vi "ion pump controller.vi"() -> ()   [LabVIEW 2010]
panel:
  out "Pressure":cluster{dbl, dbl}[](graph)
  in  "TC or AC?":u16(ring) items=["AC", "TC"]
  out "Pressure (Torr)":dbl
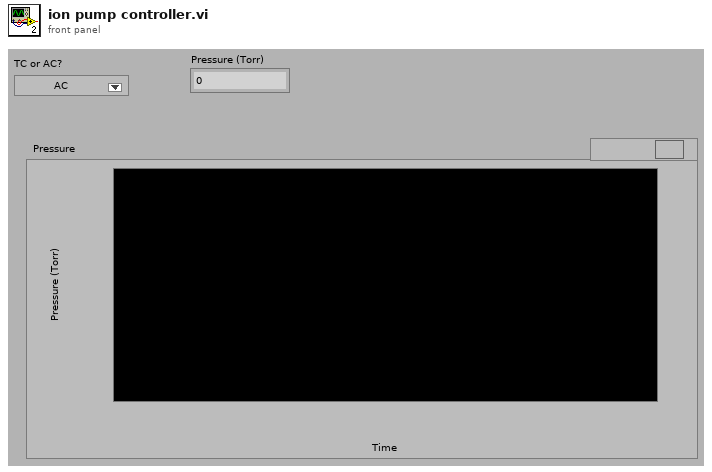
[diagram p1: front panel]
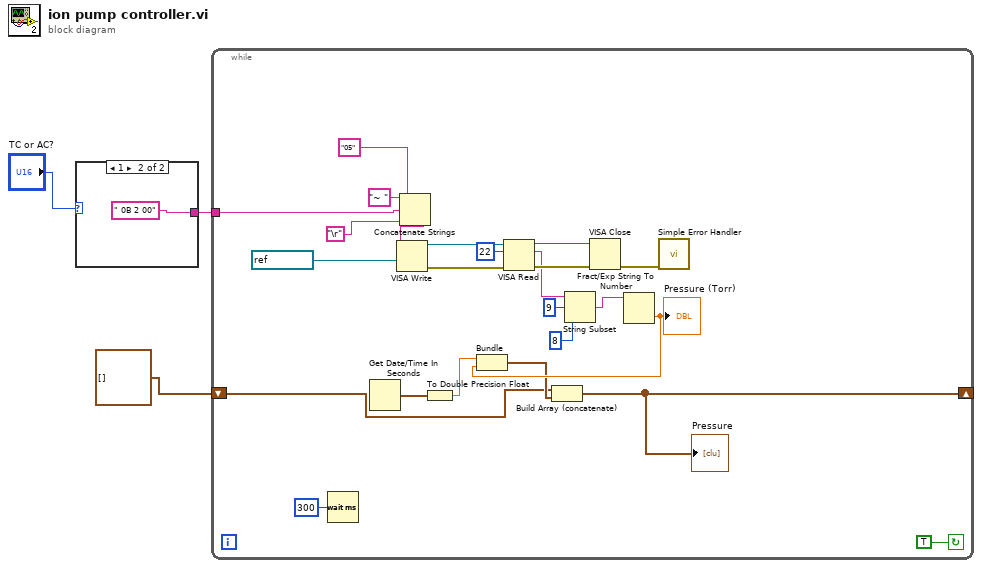
[diagram p0: block diagram]
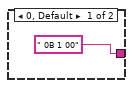
[diagram p2: hidden frame]
diagram:
  n1 = case shown="1" "TC or AC?" {
    tunnel: [" 0B 1 00" ("string") " 0B 2 00" ("string")] -> w3
    frame 0, Default {
    }
    frame 1 {
    }
  }
  n2 = while {
    tunnel: w3 -> [w18]
    shift-right: [w7] -> _
    shift-left: cluster{dbl, dbl}[] [] -> [w8]
    stop <- TRUE continue-if-true
    n3 = Wait (ms)(milliseconds to wait=u32 300) -> ()  [unwired: 1 out]
    n4 = Get Date/Time In Seconds() -> (seconds since 1Jan1904=w12:timestamp)
    n5 = Concatenate Strings("~ " ("string"), "05" ("string"), w18, "\r") -> (w29:string)
    n6 = VISA Write(VISA resource name=refnum<visa-resource-name> "COM3", write buffer=w29) -> (VISA resource name out=w27:refnum<visa-resource-name>, error out=w23:errorcluster)  [unwired: 1 in, 1 out]
    n7 = To Double Precision Float(number=w12) -> (double precision float=w11:dbl)
    n8 = VISA Read(VISA resource name=w27, byte count=u32 22, error in (no error)=w23) -> (VISA resource name out=w26:refnum<visa-resource-name>, read buffer=w17:string, error out=w24:errorcluster)  [unwired: 1 out]
    n9 = String Subset(string=w17, offset (0)=9, length (rest)=8 ("length (rest)")) -> (substring=w14:string)
    n10 = VISA Close(VISA resource name=w26, error in (no error)=w24) -> (error out=w25:errorcluster)
    n11 = Fract/Exp String To Number(string=w14) -> (number=w10:dbl)  [unwired: 3 in, 1 out]
    "Pressure (Torr)" <- w10
    n12 = Bundle(w11, w10) -> (w9:cluster{dbl, dbl})  [unwired: 1 in]
    n13 = Build Array (concatenate)(w8, w9) -> (w7:cluster{dbl, dbl}[])
    "Pressure" <- w7
    n14 = call <vilib>:"Simple Error Handler.vi"("error in (no error)"=w25) -> ()  [unwired: 4 in, 5 out]
  }
